vi "找目标.vi"(8 "error in (no error)":errorcluster, 9 "Matches (pixel)":T2(array[cluster]), 10 "temp":T1, 11 "Image":T1) -> (0 "error out":errorcluster, 2 "line":T3, 3 "目标点":cluster{i32, dbl})   [LabVIEW 2014]
uses:
  <vilib>/vision/Image Controls.llb/IMAQ Image.ctl
panel:
  out "Image Pixels (U8)":u8[][](array[numeric])
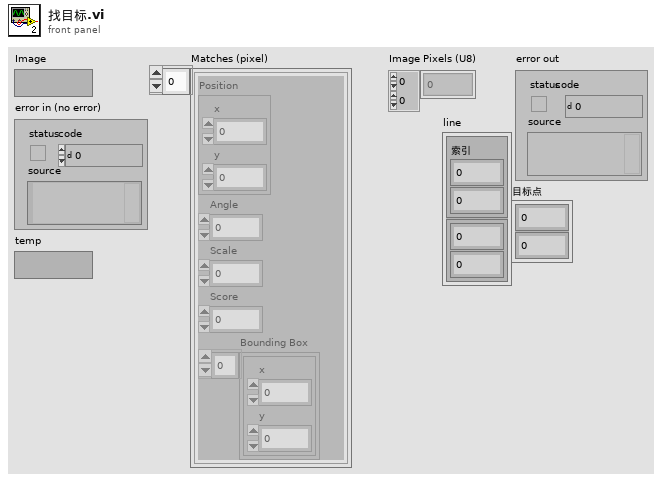
[diagram p1: front panel]
types:
  T1 = typedef "IMAQ Image.ctl" = refnum<image>
  T2 = cluster{"Position":cluster{"x":sgl, "y":sgl}, "Angle":sgl, "Scale":sgl, "Score":sgl, "Bounding Box":cluster{"x":sgl, "y":sgl}[]}[]
  T3 = cluster{cluster{"索引":i32, dbl}, cluster{i32, dbl}}
  T4 = cluster{"Position":cluster{"x":sgl, "y":sgl}, "Angle":sgl, "Scale":sgl, "Score":sgl, "Bounding Box":cluster{"x":sgl, "y":sgl}[]}
  T5 = cluster{cluster{dbl, "索引":i32}, cluster{dbl, i32}}
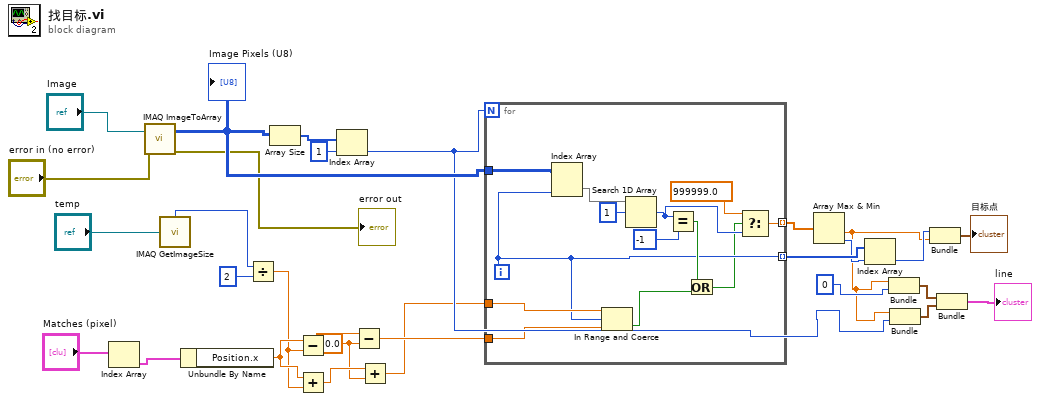
[diagram p0: block diagram]
diagram:
  w3 = 10.0 ("y")
  n1 = Index Array(array="Matches (pixel)") -> (element=w10:T4)  [unwired: 1 in]
  n2 = call "IMAQ ImageToArray"("error in (no error)"="error in (no error)", "Image"="Image") -> ("error out"=→"error out":errorcluster, "Image Pixels (U8)"=w27:u8[][])  [unwired: 2 in, 3 out]
  "Image Pixels (U8)" <- w27
  n3 = call "IMAQ GetImageSize"("Image"="temp") -> ("X Resolution"=w9:i32)  [unwired: 3 in, 2 out]
  n4 = Unbundle By Name(w10) -> ("Position.x"=w7:sgl)
  n5 = Divide(x=w9, y=2) -> (x/y=w6:dbl)
  n6 = Array Size(array=w27) -> (size(s)=w26:i32[])
  n7 = Subtract(x=w7, y=w6) -> (x-y=w5:dbl)
  n8 = Add(x=w7, y=w6) -> (x+y=w4:dbl)
  n9 = Index Array(array=w26, index=1 ("索引")) -> (element=w13:i32)
  n10 = Subtract(x=w5, y=w3) -> (x-y=w2:dbl)
  n11 = Add(x=w4, y=w3) -> (x+y=w1:dbl)
  n12 = for {
    N: w13 -> [_]
    tunnel: w27 -> [w42]
    tunnel: [w37] -> w24 mode=indexing
    tunnel: [w32] -> w19 mode=indexing
    tunnel: w2 -> [w34]
    tunnel: w1 -> [w33]
    i -> [w32]
    n13 = Index Array(array=w42, index (col)=w32) -> (element=w36:u8[])  [unwired: 1 in]
    n14 = In Range and Coerce(upper limit=w33, x=w32, lower limit=w34) -> (In Range?=w31:bool)  [unwired: 1 out]
    n15 = Search 1D Array(1D array=w36, element=u8 1 ("元素")) -> (index of element=w38:i32)  [unwired: 1 in]
    n16 = Equal?(x=w38, y=-1) -> (x = y?=w35:bool)
    n17 = Or(x=w35, y=w31) -> (x .or. y?=w30:bool)
    n18 = Select(t=999999.0, s=w30, f=w38) -> (s? t:f=w37:dbl)
  }
  n19 = Array Max & Min(array=w24) -> (min value=w14:dbl, min index (indices)=w18:i32)  [unwired: 2 out]
  n20 = Index Array(array=w19, index=w18) -> (element=w17:i32)
  n21 = Bundle(w14, "索引"=0) -> (w23:cluster{dbl, "索引":i32})  [unwired: 1 in]
  n22 = Bundle(w14, w13) -> (w22:cluster{dbl, i32})  [unwired: 1 in]
  n23 = Bundle(w17, w14) -> (→"目标点":cluster{i32, dbl})  [unwired: 1 in]
  n24 = Bundle(w23, w22) -> (→"line":T5)  [unwired: 1 in]
